vi "InvMP_Host.vi"() -> ()   [LabVIEW 2019]
uses:
  <vilib>/rvi/interface/nirviMethod/nirviMethod.xnode
  <vilib>/rvi/errors/niLvFpgaMergeErrorWithErrorCode.vi
  <vilib>/rvi/interface/nirviReadWriteControl/nirviReadWriteControl.xnode
  <vilib>/rvi/interface/Simulation/niFpgaSimulationCallBeginRW.vi
  <vilib>/rvi/errors/niLvFpgaAdjustHostInterfaceError.vi
  <vilib>/Utility/file.llb/Write Delimited Spreadsheet (DBL).vi
  <vilib>/Analysis/NI_AALBase.lvlib
  <vilib>/Analysis/baseanly.llb/Mean (DBL).vi
  <vilib>/FPGAPlugInAG/Dynamic/niLvFpga_Reset_Dynamic.vi
  <vilib>/FPGAPlugInAG/Dynamic/niLvFpga_Run_Dynamic.vi
  <vilib>/rvi/interface/nirviCloseFPGA/nirviCloseFPGA.xnode
  <vilib>/rvi/interface/nirviOpenFPGA/nirviOpenFPGA.xnode
  <vilib>/FPGAPlugInAG/Dynamic/niLvFpga_ConfigureFifo_Dynamic.vi
  <vilib>/FPGAPlugInAG/Dynamic/niLvFpga_StartFifo_Dynamic.vi
  <vilib>/FPGAPlugInAG/Dynamic/niLvFpga_ReadFifo_Dynamic.vi
  <vilib>/FPGAPlugInAG/Dynamic/niLvFpga_StopFifo_Dynamic.vi
  <vilib>/FPGAPlugInAG/Dynamic/niLvFpga_Close_Dynamic.vi
panel:
  in  "time to reach init point":sgl=75.0
  in  "Fiting Control":enum32{"Fitting Control", "Fitting Errors"}(tab)
  out "signal\n offset_X":sgl=5.0
  in  "Fit?":bool
  out "best fit parameters":sgl[](array[numeric])=[0.56758124, 58.059307, 1.2633921, 128.14603, 862.4223, 56080.08]
  out "residue":dbl
  in  "initial\nparameters":dbl[](array[numeric])=[0.0, 65.0, 0.0, -747.0, 30000.0, 300000.0, 0.0]
  in  "Offset":sgl=5.0
  out "Fitting in \nprogress":bool
  in  "Cal px/V":dbl=93.535 format="%#_13g"
  out "Pos array":sgl[](array[numeric])
  out "Volt":sgl[](array[numeric])
  out "error out":errorcluster
  out "smoothing error":i32
  in  "Calibration":T1={"K0"=0.0, "K1"=1.0, "K2"=0.0, "K3"=0.0, "K4"=0.0, "K5"=0.0}
  in  "Use Cal?":bool=TRUE
  in  "V_offset":sgl
  in  "Bias":sgl=0.00019
  in  "Xmin":sgl=-1.0
  in  "Fmax":sgl=30000.0
  in  "Xmax":sgl=2.0
  in  "cdfnorm":sgl=1.0
  out "num of protocols":sgl=5153.0
  in  "Calibration ON/OFF":bool=TRUE
  in  "Xoffset":sgl=0.00147
  in  "Yoffset":sgl=-0.00294
  in  "sum_offset":sgl=-0.0068
  out "Xpot":sgl=-0.92444557 format="%.2f"
  in  "wait time":u8=80
  in  "Temp":i8(ring)=1 items=["Cold", "Warm", "Hot"]
  in  "?":u16(ring) items=["No FB", "FB"]
  in  "DW":cluster{"xm":sgl, "Eb":sgl, "Tau":sgl, "dE":sgl}={"xm"=0.5, "Eb"=0.005, "Tau"=70.0, "dE"=0.001} {"dE" format="%#_3g"}
  in  "DL_Y":dbl=2.5 format="%#_13g"
  in  "TL_Y":dbl=2.5 format="%#_13g"
  in  "STOP":bool
  in  "FB time":u32=10
  in  "Triangle wave":T2={"signal offset_X"=5.0, "Scale X"=0.0, "signal offset_Y"=5.0, "Scale Y"=0.0, "Phase Shift"=40}
  in  "Elements":u32=100000
  in  "Data length":dbl=750.0
  out "Done saving":bool
  out "?":dbl=-23.0
  in  "Save Data":bool
  in  "mobX(px/V)":sgl=1.0
  in  "1/Xcali":sgl=1.0
  in  "DX":sgl=53.374
  out "Feedback Loop time":sgl=10.0 format="%.2f"
  out "Underflow":bool
  out "Fx out/Xcorr":sgl=5.0
  out "X":waveform(dbl)(graph)={"t0"=timestamp(0 s since 1904-01-01), "dt"=9.999999747378752e-06, "Y"=array[100000 elements]}
  out "Y":waveform(dbl)(graph)={"t0"=timestamp(0 s since 1904-01-01), "dt"=9.999999747378752e-06, "Y"=array[100000 elements]}
  out "Sum":waveform(dbl)(graph)={"t0"=timestamp(0 s since 1904-01-01), "dt"=9.999999747378752e-06, "Y"=array[100000 elements]}
  in  "Reaverage PS":bool
  out "meanX":dbl=0.17730553089997972 format="%0.5f"
  in  "Xmean":sgl
  out "PSX":dynamicdata(graph)=[{"t0"=timestamp(0 s since 1904-01-01), "dt"=1.0000000252621255, "Y"=array[50000 elements], "attributes"=variant("NI_ChannelName"=variant(string "PSD"))}]
  out "PSY":dynamicdata(graph)=[{"t0"=timestamp(0 s since 1904-01-01), "dt"=1.0000000252621255, "Y"=array[50000 elements], "attributes"=variant("NI_ChannelName"=variant(string "PSD"))}]
  out "PSsum":dynamicdata(graph)=[{"t0"=timestamp(0 s since 1904-01-01), "dt"=1.0000000252621255, "Y"=array[50000 elements], "attributes"=variant("NI_ChannelName"=variant(string "PSD"))}]
  out "Saveloop":u32
  in  "Feedback parameters":T3={"SP_QPDX"=0.0, "alpha"=0.1, "ktrap"=46.2263, "alphacounterX"=0.0228223}
  in  "TW freq":dbl=1.0
  in  "Normalize signal":bool=TRUE
  out "meanY":dbl=0.06301697970006614 format="%0.5f"
  out "meanZ":dbl=0.5391900868940354 format="%0.4f"
  out "?":errorcluster
  in  "file path (dialog if empty)":path=path "C:/Users/Diffusivity/Desktop/Inverse_Mpemba_starting June16/09-09-2020/t.txt"
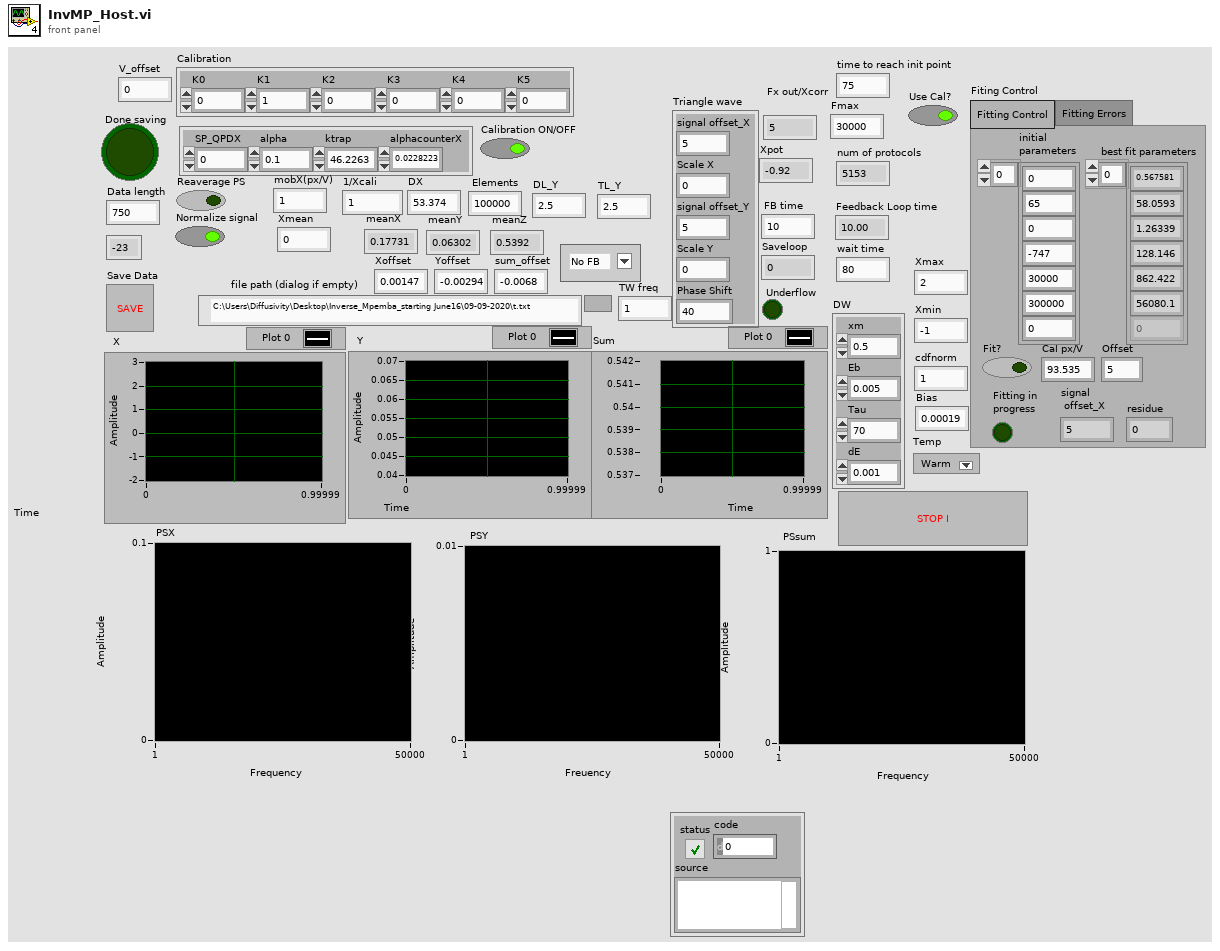
[diagram p1: front panel]
types:
  T1 = cluster{"K0":sgl, "K1":sgl, "K2":sgl, "K3":sgl, "K4":sgl, "K5":sgl}
  T2 = cluster{"signal offset_X":sgl, "Scale X":sgl, "signal offset_Y":sgl, "Scale Y":sgl, "Phase Shift":u32}
  T3 = cluster{"SP_QPDX":sgl, "alpha":sgl, "ktrap":sgl, "alphacounterX":sgl}
  T4 = cluster{"signal offset_X":sgl, "Scale X":sgl, "signal offset_Y":sgl, "Scale Y":sgl, u32}
  T5 = cluster{"[0]":sgl, "[1]":sgl, "[2]":sgl, "[3]":sgl, "[4]":sgl, "[5]":sgl}
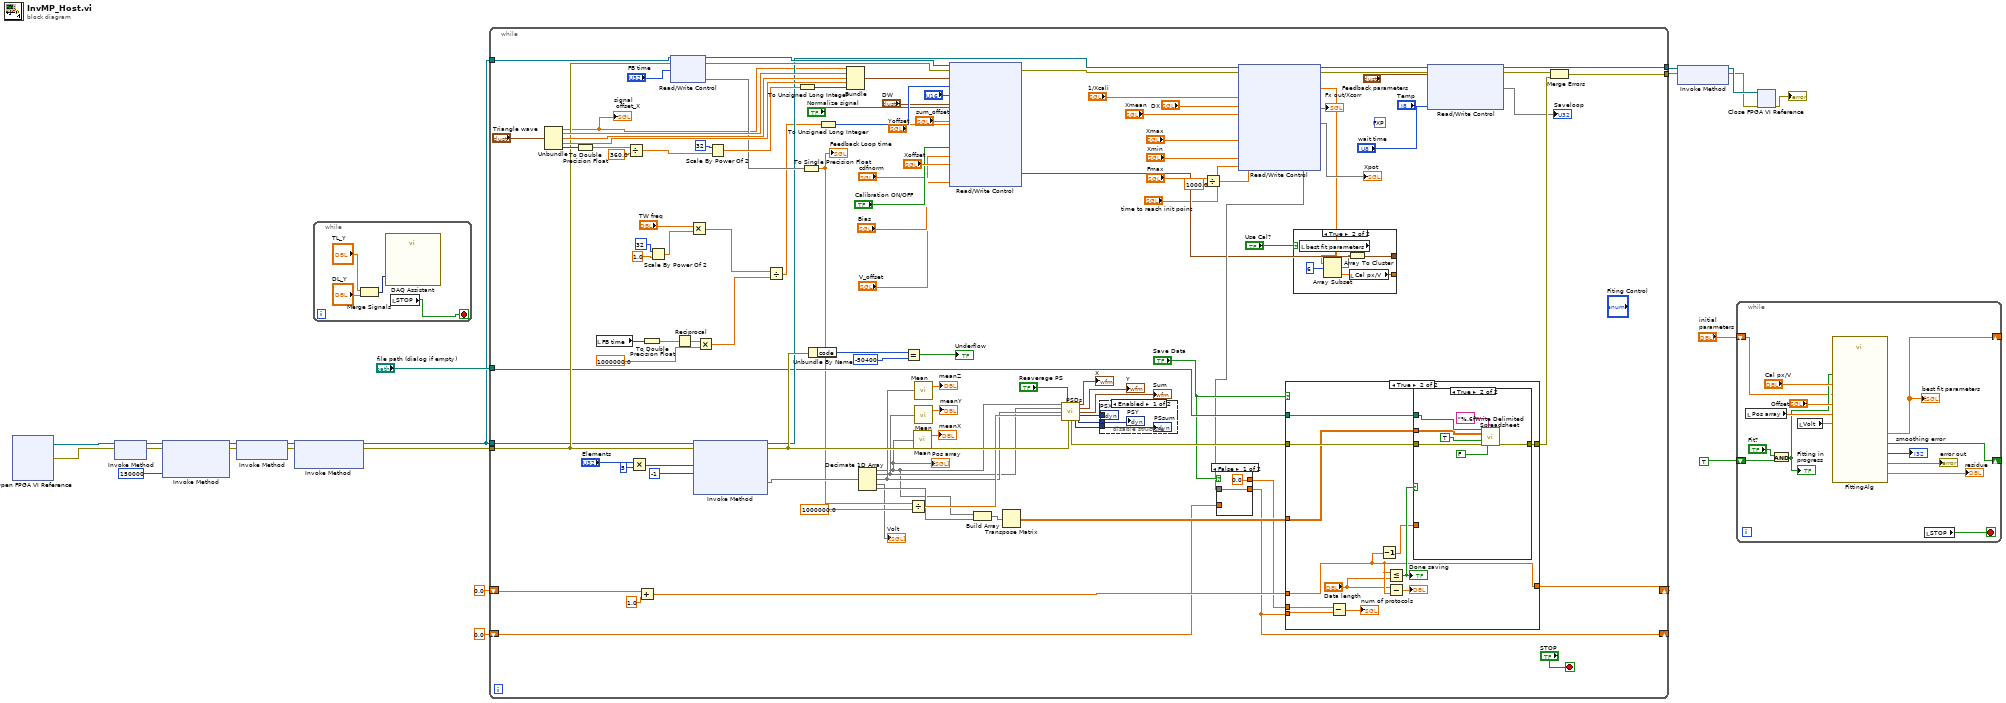
[diagram p0: block diagram]
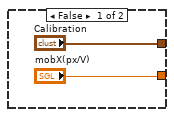
[diagram p2: hidden frame]
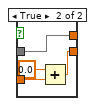
[diagram p3: hidden frame]
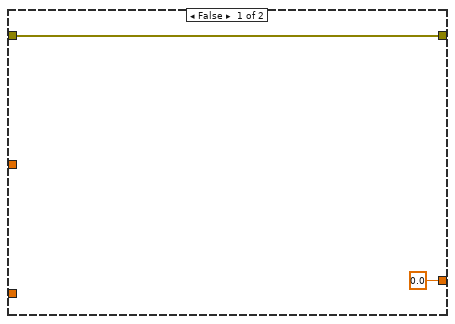
[diagram p5: hidden frame]
diagram:
  n1 = xnode "Open FPGA VI Reference"() -> ("FPGA VI Reference Out"=w4:refnum<k20>, "error out"=w3:errorcluster)  [unwired: 2 in]
  n2 = xnode "Invoke Method"("FPGA VI Reference In"=w4, "error in"=w3) -> ("FPGA VI Reference Out"=w11:refnum<k20>, "error out"=w10:errorcluster)
  n3 = xnode "Invoke Method"("FPGA VI Reference In"=w11, "error in"=w10, "Requested Depth"=u32 150000) -> ("FPGA VI Reference Out"=w16:refnum<k20>, "error out"=w15:errorcluster)  [unwired: 1 out]
  n4 = xnode "Invoke Method"("FPGA VI Reference In"=w16, "error in"=w15) -> ("FPGA VI Reference Out"=w18:refnum<k20>, "error out"=w17:errorcluster)
  n5 = xnode "Invoke Method"("FPGA VI Reference In"=w18, "error in"=w17) -> ("FPGA VI Reference Out"=w14:refnum<k20>, "error out"=w13:errorcluster)  [unwired: 1 in]
  n6 = while {
    stop <- w22 stop-if-true
    n7 = Merge Signals("TL_Y", "DL_Y") -> (w25:dynamicdata)
    n8 = call "DAQ Assistant"("data"=w25) -> ()  [unwired: 17 in, 2 out]
    n9 = local read "STOP"() -> (w22:bool)
  }
  n10 = while {
    tunnel: w14 -> [w110]
    tunnel: w13 -> [w111]
    tunnel: "file path (dialog if empty)" -> [w78]
    tunnel: [w103] -> w20
    tunnel: [w116] -> w19
    tunnel: w14 -> [w98]
    shift-right: [w107] -> _
    shift-left: 0.0 -> [w106]
    shift-right: [w44] -> _
    shift-left: sgl 0.0 ("num of cycles") -> [w46]
    stop <- "STOP" stop-if-true
    (unwired) fxp<+,8,7> 50.0 ("Fmax")
    n11 = Unbundle("Triangle wave") -> ("signal offset_X"=w27:sgl, "Scale X"=w120:sgl, "signal offset_Y"=w119:sgl, "Scale Y"=w118:sgl, "Phase Shift"=w121:u32)
    "signal\n offset_X" <- w27
    n12 = To Double Precision Float(number=w121) -> (double precision float=w127:dbl)
    n13 = local read "FB time"() -> (w68:u32)
    n14 = Divide(x=w127, y=360.0) -> (x/y=w125:dbl)
    n15 = Multiply(x="Elements", y=u32 5) -> (x*y=w112:u32)
    n16 = Add(x=w106, y=1.0) -> (x+y=w108:dbl)
    n17 = To Double Precision Float(number=w68) -> (double precision float=w69:dbl)
    n18 = Scale By Power Of 2(n=i16 32, x=1.0) -> (x*2^n=w73:dbl)
    n19 = xnode "Read/Write Control"("FPGA VI Reference In"=w110, "error in"=w111, "FB Time"="FB time") -> ("FPGA VI Reference Out"=w132:refnum<k20>, "error out"=w99:errorcluster, "FB Time"=w97)
    n20 = Reciprocal(x=w69) -> (1/x=w70:dbl)
    n21 = Multiply(x="TW freq", y=w73) -> (x*y=w66:dbl)
    n22 = xnode "Invoke Method"("FPGA VI Reference In"=w98, "error in"=w111, "Number of Elements"=w112, "Timeout (ms)"=-1) -> ("FPGA VI Reference Out"=w80:refnum<k20>, "error out"=w95:errorcluster, "Data"=w90:void[])  [unwired: 1 out]
    n23 = Multiply(x=w70, y=1000000.0) -> (x*y=w65:dbl)
    n24 = Scale By Power Of 2(n=i16 32, x=w125) -> (x*2^n=w123:dbl)
    n25 = Divide(x=w66, y=w65) -> (x/y=w64:dbl)
    n26 = To Unsigned Long Integer(number=w123) -> (unsigned 32bit integer=w117:u32)
    n27 = To Single Precision Float(number=w97) -> (single precision float=w75:sgl)
    "Feedback Loop time" <- w75
    n28 = Unbundle By Name(w95) -> ("code"=w115:i32)
    n29 = To Unsigned Long Integer(number=w64) -> (unsigned 32bit integer=w63:u32)
    n30 = Bundle("signal offset_X"=w27, "Scale X"=w120, "signal offset_Y"=w119, "Scale Y"=w118, w117) -> (w76:T4)  [unwired: 1 in]
    n31 = Decimate 1D Array(w90) -> (w29:void[], w52:void[], w56:void[], →"Volt":void[], w57:void[])
    "Pos array" <- w29
    n32 = Equal?(x=w115, y=-50400) -> (x = y?=→"Underflow":bool)
    n33 = Divide(x=w75, y=sgl 1000000.0) -> (x/y=w58:sgl)
    n34 = call-poly <vilib>:"Mean.vi"("X"=w29) -> ("mean"=→"meanX":dbl)  [unwired: 1 out]
    n35 = call-poly <vilib>:"Mean.vi"("X"=w56) -> ("mean"=→"meanZ":dbl)  [unwired: 1 out]
    n36 = call-poly <vilib>:"Mean.vi"("X"=w52) -> ("mean"=→"meanY":dbl)  [unwired: 1 out]
    n37 = Build Array(w29, w57) -> (w101:void[])
    n38 = Transpose Matrix(1:w101) -> (0:w130:dbl[][])
    n39 = call "PSDs.vi"("X"=w29, "averaging done"="Reaverage PS", "Y"=w52, "sum"=w56, "dt"=w58, "error in (no error)"=w95) -> ("X"=→"X":waveform(dbl), "Y"=→"Y":waveform(dbl), "Sum"=→"Sum":waveform(dbl), "PSDX"=w86:dynamicdata, "error out"=w94:errorcluster, "PSDsum"=w84:dynamicdata, "PSDY"=w85:dynamicdata)  [unwired: 3 in]
    n40 = disable-structure shown="Enabled" {
      disable-tunnel: w86 -> [w150 _]
      disable-tunnel: w85 -> [w149 _]
      disable-tunnel: w84 -> [w148 _]
      frame Enabled {
        "PSX" <- w150
        "PSY" <- w149
        "PSsum" <- w148
      }
      frame Disabled {
      }
    }
    n41 = Divide(x="Fmax", y=sgl 1000.0) -> (x/y=w37:sgl)
    n42 = case shown="True" "Use Cal?" {
      tunnel: ["Calibration" w141] -> w31
      tunnel: ["mobX(px/V)" w138] -> w30
      frame False {
      }
      frame True {
        n43 = local read "best fit parameters"() -> (w137:sgl[])
        n44 = Array Subset(array=w137, length=6) -> (w139:sgl[])  [unwired: 1 in]
        n45 = Array To Cluster(array=w139) -> (cluster=w141:T5)
        n46 = local read "Cal px/V"() -> (w138:dbl)
      }
    }
    n47 = xnode "Read/Write Control"("FPGA VI Reference In"=w132, "error in"=w99, "Triangle wave"=w76, "Frequency"=w63, "Enum"="?", "DW"="DW", "Normalize signal"="Normalize signal", "sum_offset"="sum_offset", "Yoffset"="Yoffset", "Xoffset"="Xoffset", "Calibration ON/OFF"="Calibration ON/OFF", "cdfnorm"="cdfnorm", "Bias"="Bias", "Calibration"=w31, "V_offset"="V_offset") -> ("error out"=w79:errorcluster)  [unwired: 1 out]
    n48 = xnode "Read/Write Control"("FPGA VI Reference In"=w80, "error in"=w79, "MobX(px/V)"=w30, "1/Xcali"="1/Xcali", "DX"="DX", "Xmean"="Xmean", "Xmax"="Xmax", "Fmax"=w37, "Xmin"="Xmin", "time to reach init point"="time to reach init point") -> ("FPGA VI Reference Out"=w105:refnum<k20>, "error out"=w104:errorcluster, "Fx out/Xcorr"=→"Fx out/Xcorr", "Xpot"=→"Xpot", "num of cycles"=w42)
    n49 = case shown="False" "Save Data" {
      tunnel: w42 -> [w143 w144]
      tunnel: [w143 w145] -> w44
      tunnel: w46 -> [_ w146]
      tunnel: [sgl 0.0 ("num of cycles") w144] -> w45
      frame False {
      }
      frame True {
        n50 = Add(x=sgl 0.0 ("num of cycles"), y=w146) -> (x+y=w145:sgl)
      }
    }
    n51 = case shown="True" "Save Data" {
      tunnel: w130 -> [_ w159]
      tunnel: w78 -> [_ w164]
      tunnel: w94 -> [w152 w163]
      tunnel: [w152 w162] -> w129
      tunnel: w108 -> [_ w158]
      tunnel: [0.0 w158] -> w107
      tunnel: w45 -> [_ w155]
      tunnel: w44 -> [_ w154]
      frame False {
      }
      frame True {
        n52 = Subtract(x=w155, y=w154) -> (x-y=→"num of protocols":sgl)
        n53 = Decrement(x=w158) -> (x-1=w157:dbl)
        n54 = Less Or Equal?(x=w158, y="Data length") -> (x <= y?=w161:bool)
        "Done saving" <- w161
        n55 = Subtract(x="Data length", y=w158) -> (x-y=→"?":dbl)
        n56 = case shown="True" w161 {
          tunnel: w159 -> [_ w166]
          tunnel: w164 -> [_ w167]
          tunnel: w163 -> [w165 w170]
          tunnel: [w165 w169] -> w162
          tunnel: w157 -> [_ _]
          frame False {
          }
          frame True {
            n57 = call-poly <vilib>:"Write Delimited Spreadsheet.vi"("file path (dialog if empty)"=w167, "format (%.3f)"="%.6f", "2D data"=w166, "append to file? (new file:F)"=TRUE, "error in (no error)"=w170, "transpose? (no:F)"=FALSE) -> ("error out"=w169:errorcluster)  [unwired: 8 in, 1 out]
          }
        }
      }
    }
    n58 = xnode "Read/Write Control"("FPGA VI Reference In"=w105, "error in"=w104, "Feedback parameters"="Feedback parameters", "Temp"="Temp", "wait time"="wait time") -> ("FPGA VI Reference Out"=w103:refnum<k20>, "error out"=w102:errorcluster, "Saveloop"=→"Saveloop")
    n59 = Merge Errors(w102, w129) -> (w116:errorcluster)
  }
  n60 = xnode "Invoke Method"("FPGA VI Reference In"=w20, "error in"=w19) -> ("FPGA VI Reference Out"=w9:refnum<k20>, "error out"=w8:errorcluster)
  n61 = while {
    shift-right: [w178] -> _
    shift-left: TRUE -> [w179]
    shift-right: [w174] -> _
    shift-left: "initial\nparameters" -> [w173]
    stop <- w185 stop-if-true
    n62 = local read "Pos array"() -> (w184:sgl[])
    n63 = And(x="Fit?", y=w179) -> (x .and. y?=w177:bool)
    "Fitting in \nprogress" <- w177
    n64 = local read "Volt"() -> (w183:sgl[])
    n65 = call "FittingAlg.vi"("Pos"=w184, "Cal px/V"="Cal px/V", "initial parameters"=w173, "Volt"=w183, "Boolean in"=w177, "Offset"="Offset") -> ("error"=→"smoothing error":i32, "best fit parameters"=w174:dbl[], "Boolean out"=w178:bool, "residue"=→"residue":dbl, "error out"=→"error out":errorcluster)  [unwired: 5 in]
    "best fit parameters" <- w174
    n66 = local read "STOP"() -> (w185:bool)
  }
  n67 = xnode "Close FPGA VI Reference"("FPGA VI Reference In"=w9, "error in"=w8) -> ("error out"=→"?":errorcluster)
